vi "Get ID.vi"(8 "error in (no error)":errorcluster, 11 "Driver in":refnum<class "Driver.lvclass">) -> (0 "error out":errorcluster, 2 "ID_DEVICE":string, 3 "Driver out":refnum<class "Driver.lvclass">)   [LabVIEW 2023, in "Driver.lvlib" / "Driver.lvclass"]
uses:
  Driver.lvclass
  Driver.lvclass/Driver.ctl
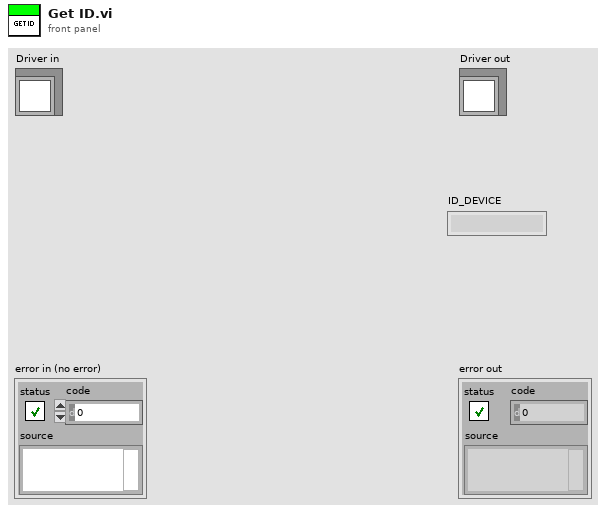
[diagram p1: front panel]
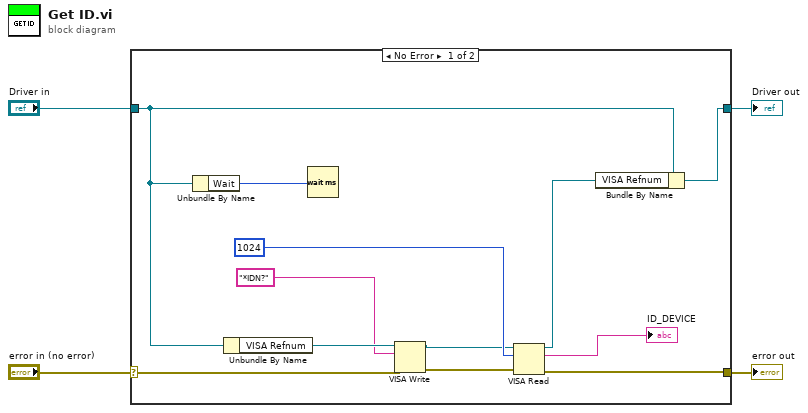
[diagram p0: block diagram]
diagram:
  n1 = case shown="No Error" "error in (no error)" {
    selector: "error in (no error)" -> [w16 w18]
    tunnel: [w10 w18] -> w3
    tunnel: [w7 w17] -> w1
    tunnel: "Driver in" -> [w6 w17]
    frame No Error {
      n2 = Unbundle By Name(w6) -> ("Wait"=w5:u16)
      n3 = Unbundle By Name(w6) -> ("VISA Refnum"=w15:refnum<visa-resource-name>)
      n4 = Wait (ms)(milliseconds to wait=w5) -> ()  [unwired: 1 out]
      n5 = VISA Write(VISA resource name=w15, write buffer="*IDN?", error in (no error)=w16) -> (VISA resource name out=w11:refnum<visa-resource-name>, error out=w12:errorcluster)  [unwired: 1 out]
      n6 = VISA Read(VISA resource name=w11, byte count=u32 1024, error in (no error)=w12) -> (VISA resource name out=w8:refnum<visa-resource-name>, read buffer=→"ID_DEVICE":string, error out=w10:errorcluster)  [unwired: 1 out]
      n7 = Bundle By Name(cluster=w6, "VISA Refnum"=w8) -> (w7:refnum<class "Driver.lvclass">)
    }
    frame Error {
    }
  }
  "error out" <- w3
  "Driver out" <- w1
